vi "close connection.vi"(8 "error in (no error)":errorcluster, 11 "MB_TCP in":refnum<class "MB_TCP.lvclass">) -> (0 "error out":errorcluster, 3 "MB_TCP out":refnum<class "MB_TCP.lvclass">)   [LabVIEW 2021, in "MB_TCP.lvclass"]
uses:
  MB_TCP.lvclass
  MB_TCP.lvclass/MB_TCP.ctl
  NI_modbus_upd/TCP/TCP.lvclass/TCP.ctl
  NI_modbus_upd/TCP/TCP.lvclass
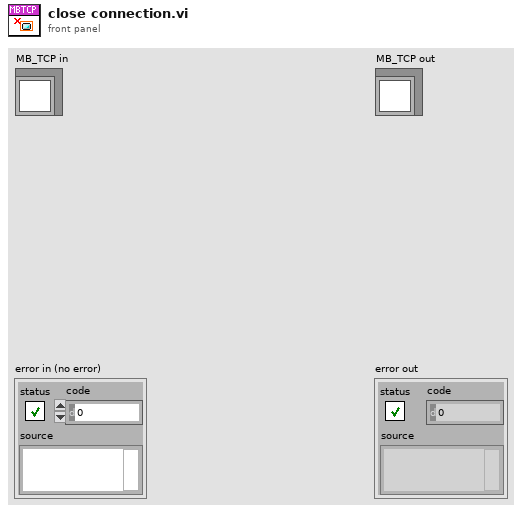
[diagram p1: front panel]
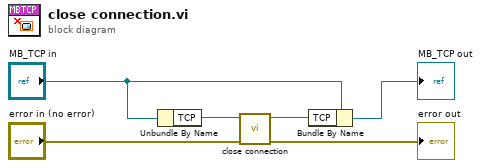
[diagram p0: block diagram]
diagram:
  n1 = Unbundle By Name("MB_TCP in") -> ("TCP"=w6:refnum<class "TCP.lvclass">)
  n2 = call "close connection.vi"("error in (no error)"="error in (no error)", "TCP in"=w6) -> ("error out"=→"error out":errorcluster, "TCP out"=w2:refnum<class "TCP.lvclass">)  [unwired: 8 in]
  n3 = Bundle By Name(cluster="MB_TCP in", "TCP"=w2) -> (→"MB_TCP out":refnum<class "MB_TCP.lvclass">)
